vi "Unregister Item.vi"(6 "Remove Dependencies?":bool, 8 "error in (no error)":errorcluster, 10 "Node":refnum<class "UniqueName.lvclass">, 11 "Registry in":refnum<data-value>) -> (0 "error out":errorcluster, 1 "Dependencies removed":string[](array[string]), 2 "Fully Qualified Name":string, 3 "Registry":refnum<data-value>)   [LabVIEW 2013, in "UniqueName.lvlib" / "NameRegistry.lvclass"]
uses:
  NameRegistry.lvclass
  UniqueNameClass/UniqueName.lvclass
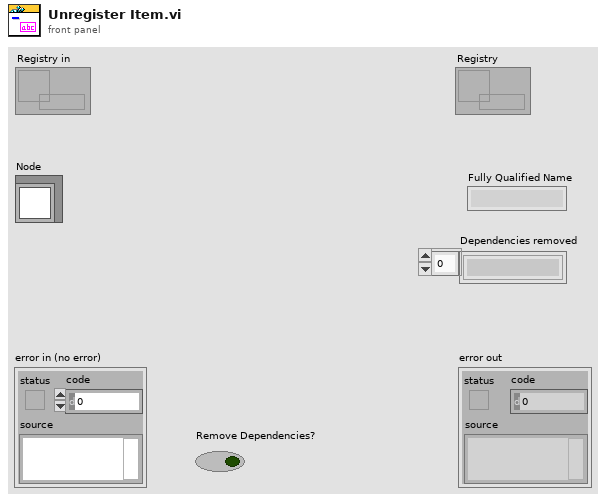
[diagram p1: front panel]
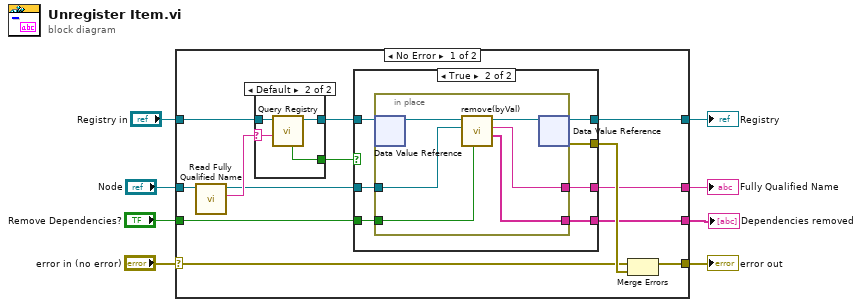
[diagram p0: block diagram]
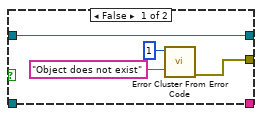
[diagram p2: hidden frame]
diagram:
  n1 = case shown="No Error" "error in (no error)" {
    selector: "error in (no error)" -> [w19 w44]
    tunnel: "Registry in" -> [w17 w45]
    tunnel: [w21 w45] -> w7
    tunnel: [w18 w44] -> w5
    tunnel: "Node" -> [w14 _]
    tunnel: [w11 _] -> w3
    tunnel: "Remove Dependencies?" -> [w10 _]
    tunnel: [w9 _] -> w1
    frame No Error {
      n2 = call "Read Fully Qualified Name.vi"("UniqueName in"=w14) -> ("Fully Qualified Name"=w13:string, "UniqueName out"=w12:refnum<class "UniqueName.lvclass">)  [unwired: 9 in]
      n3 = case shown="Default" w13 {
        selector: w13 -> [_ w41]
        tunnel: w17 -> [w39 w43]
        tunnel: [w39 w42] -> w16
        tunnel: [_ w40] -> w15
        frame "" {
        }
        frame Default {
          n4 = call "Query Registry.vi"("Search string"=w41, "Registry in"=w43) -> ("Registry"=w42:refnum<data-value>, "found?"=w40:bool)  [unwired: 5 in, 3 out]
        }
      }
      n5 = case shown="True" w15 {
        tunnel: [w25 w32] -> w21
        tunnel: [w23 w31] -> w20
        tunnel: w16 -> [w25 w30]
        tunnel: w12 -> [_ w29]
        tunnel: [_ w28] -> w11
        tunnel: w10 -> [_ w27]
        tunnel: [_ w26] -> w9
        frame False {
          n6 = call <vilib>:"Error Cluster From Error Code.vi"("error message (\"\")"="Object does not exist" ("error message (\"\")"), "error code (0)"=1) -> ("error out"=w23:errorcluster)  [unwired: 7 in]
        }
        frame True {
          n7 = in-place {
            in-place-border: w29 -> [w38]
            in-place-border: [w35] -> w28
            in-place-border: w27 -> [w34]
            in-place-border: [w33] -> w26
            n8 = in-place-dvr #1(w30) -> (w37:refnum<class "NameRegistry.lvclass">)  [unwired: 1 out]
            n9 = call "remove(byVal).vi"("Remove Dependencies?"=w34, "UniqueName in"=w38, "NameRegistry in"=w37) -> ("Dependencies removed"=w33:string[], "Fully Qualified Name"=w35:string, "NameRegistry out"=w36:refnum<class "NameRegistry.lvclass">)  [unwired: 6 in]
            n10 = in-place-dvr #1(w36) -> (w32:refnum<data-value>, w31:errorcluster)
          }
        }
      }
      n11 = Merge Errors(w19, w20) -> (w18:errorcluster)
    }
    frame Error {
    }
  }
  "error out" <- w5
  "Registry" <- w7
  "Fully Qualified Name" <- w3
  "Dependencies removed" <- w1
